vi "SMR_LabVIEW_V6.vi"() -> ()   [LabVIEW 2025]
uses:
  <vilib>/DAQmx/read.llb/DAQmx Read (Analog 1D DBL NChan 1Samp).vi
  <vilib>/DAQmx/create/channels.llb/DAQmx Create Channel (AI-Temperature-Thermocouple).vi
  <vilib>/DAQmx/create/channels.llb/DAQmx Create Channel (AI-Voltage-Basic).vi
  <vilib>/DAQmx/miscellaneous.llb/DAQmx Fill In Error Info.vi
panel:
  in  "Flow CSV Path":path
  in  "Pressure CSV Path":path
  in  "Temeprature CSV Path":path
  out "Heat Exchanger Pressure History":dbl(graph)
  out "Main Loop Pressure History":T1(graph)
  out "Heat Exchanger Temperature History":cluster{"Waveform":dbl, "Waveform":dbl}(graph)
  out "Main Loop Temeperature History":T2(graph)
  out "Overall Avg Pressure (psi)":dbl
  out "Heat Exchanger Pressure P6 (psi)":dbl
  out "Main Loop Avg Pressure (psi)":dbl
  out "Heat Exchanger Avg Temp (deg C)":dbl
  out "Main Loop Avg Temp (deg C)":dbl
  out "Raw NI9201 \nVoltage Display":T3
  out "Temperature Display":T4
  out "Pressure Display":T5
  in  "Flow Offset Correction (GPM)":dbl=-0.3
  out "Flow History":dbl(graph)
  out "Overall Pressure History":T6(graph)
  out "Overall Temperature History":T7(graph)
  out "Max Loop Pressure (psi)":dbl
  out "Overall Avg Temp (deg C)":dbl
  out "Max Loop Temp (deg C)":dbl
  out "Heat Exchanger Flow (GPM)":dbl
  in  "Loop Period (ms)":dbl=1000.0
  in  "Stop":bool
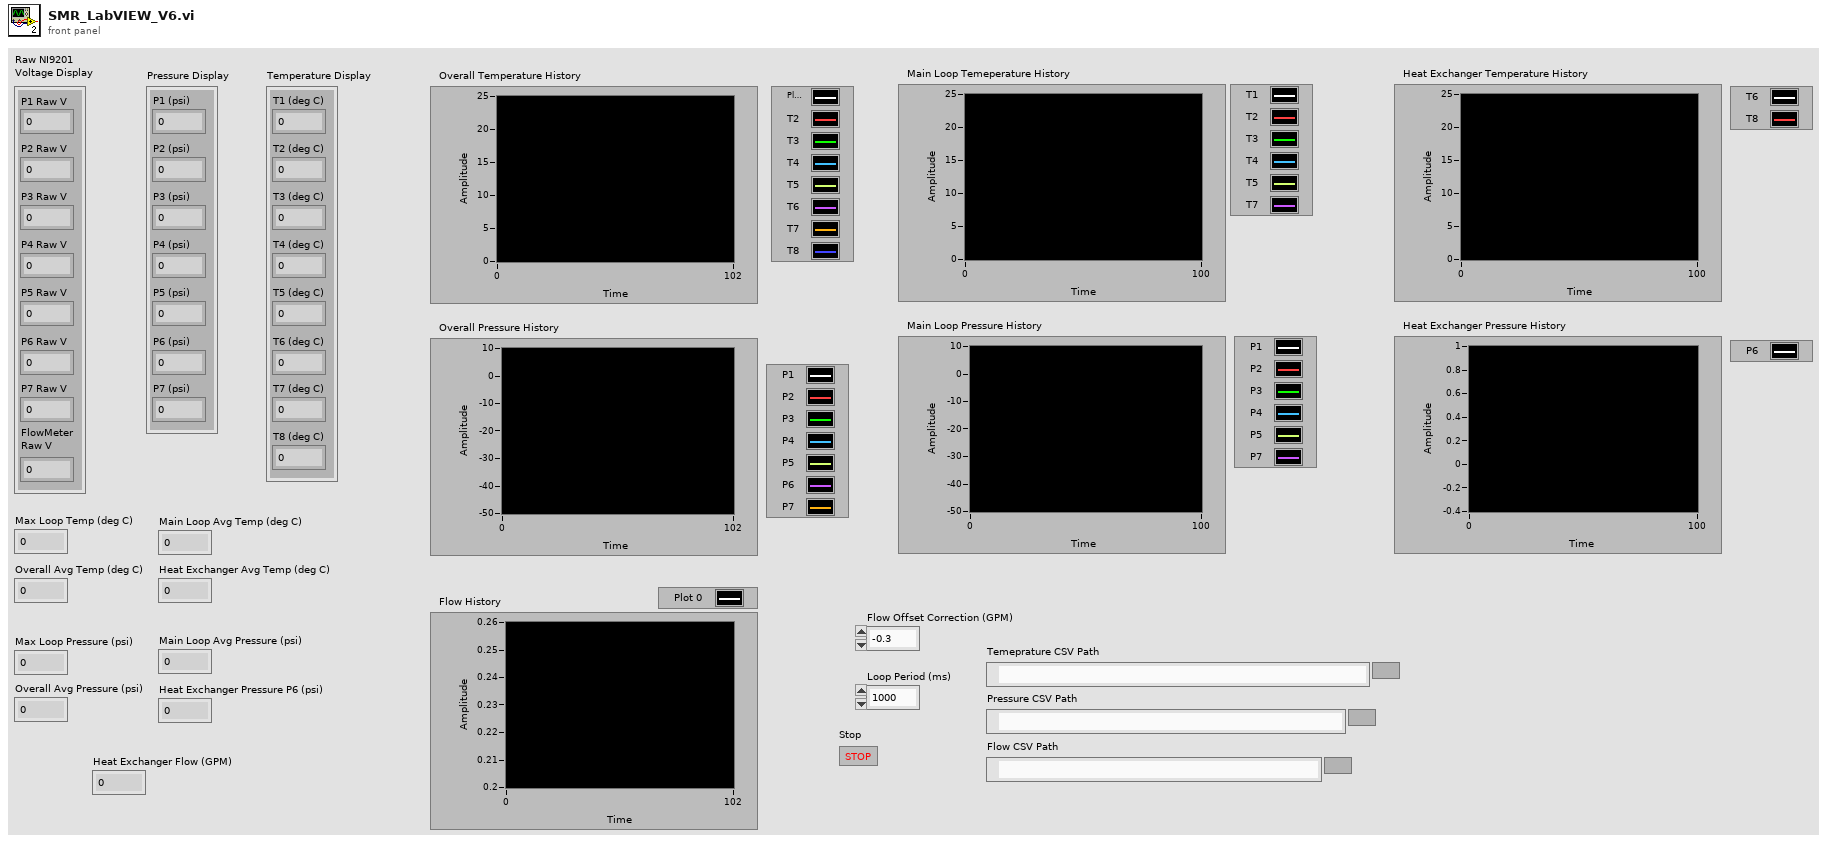
[diagram p1: front panel]
types:
  T1 = cluster{"P1":dbl, "P2":dbl, "P3":dbl, "P4":dbl, "P5":dbl, "P7":dbl}
  T2 = cluster{"Waveform":dbl, "Waveform":dbl, "Waveform":dbl, "Waveform":dbl, "Waveform":dbl, "Waveform":dbl}
  T3 = cluster{"P1 Raw V":dbl, "P2 Raw V":dbl, "P3 Raw V":dbl, "P4 Raw V":dbl, "P5 Raw V":dbl, "P6 Raw V":dbl, "P7 Raw V":dbl, "FlowMeter\nRaw V":dbl}
  T4 = cluster{"T1 (deg C)":dbl, "T2 (deg C)":dbl, "T3 (deg C)":dbl, "T4 (deg C)":dbl, "T5 (deg C)":dbl, "T6 (deg C)":dbl, "T7 (deg C)":dbl, "T8 (deg C)":dbl}
  T5 = cluster{"P1 (psi)":dbl, "P2 (psi)":dbl, "P3 (psi)":dbl, "P4 (psi)":dbl, "P5 (psi)":dbl, "P6 (psi)":dbl, "P7 (psi)":dbl}
  T6 = cluster{"P1":dbl, "P2":dbl, "P3":dbl, "P4":dbl, "P5":dbl, "P6":dbl, "P7":dbl}
  T7 = cluster{"Waveform":dbl, "Waveform":dbl, "Waveform":dbl, "Waveform":dbl, "Waveform":dbl, "Waveform":dbl, "Waveform":dbl, "Waveform":dbl}
  T8 = enum16{"open", "replace", "create", "open or create", "replace or create", "replace or create with confirmation"}
  T9 = cluster{"P1":dbl, "P2":dbl, "P3":dbl, "P4":dbl, "P5":dbl, "P6":dbl, "P7":dbl, "Flow":dbl}
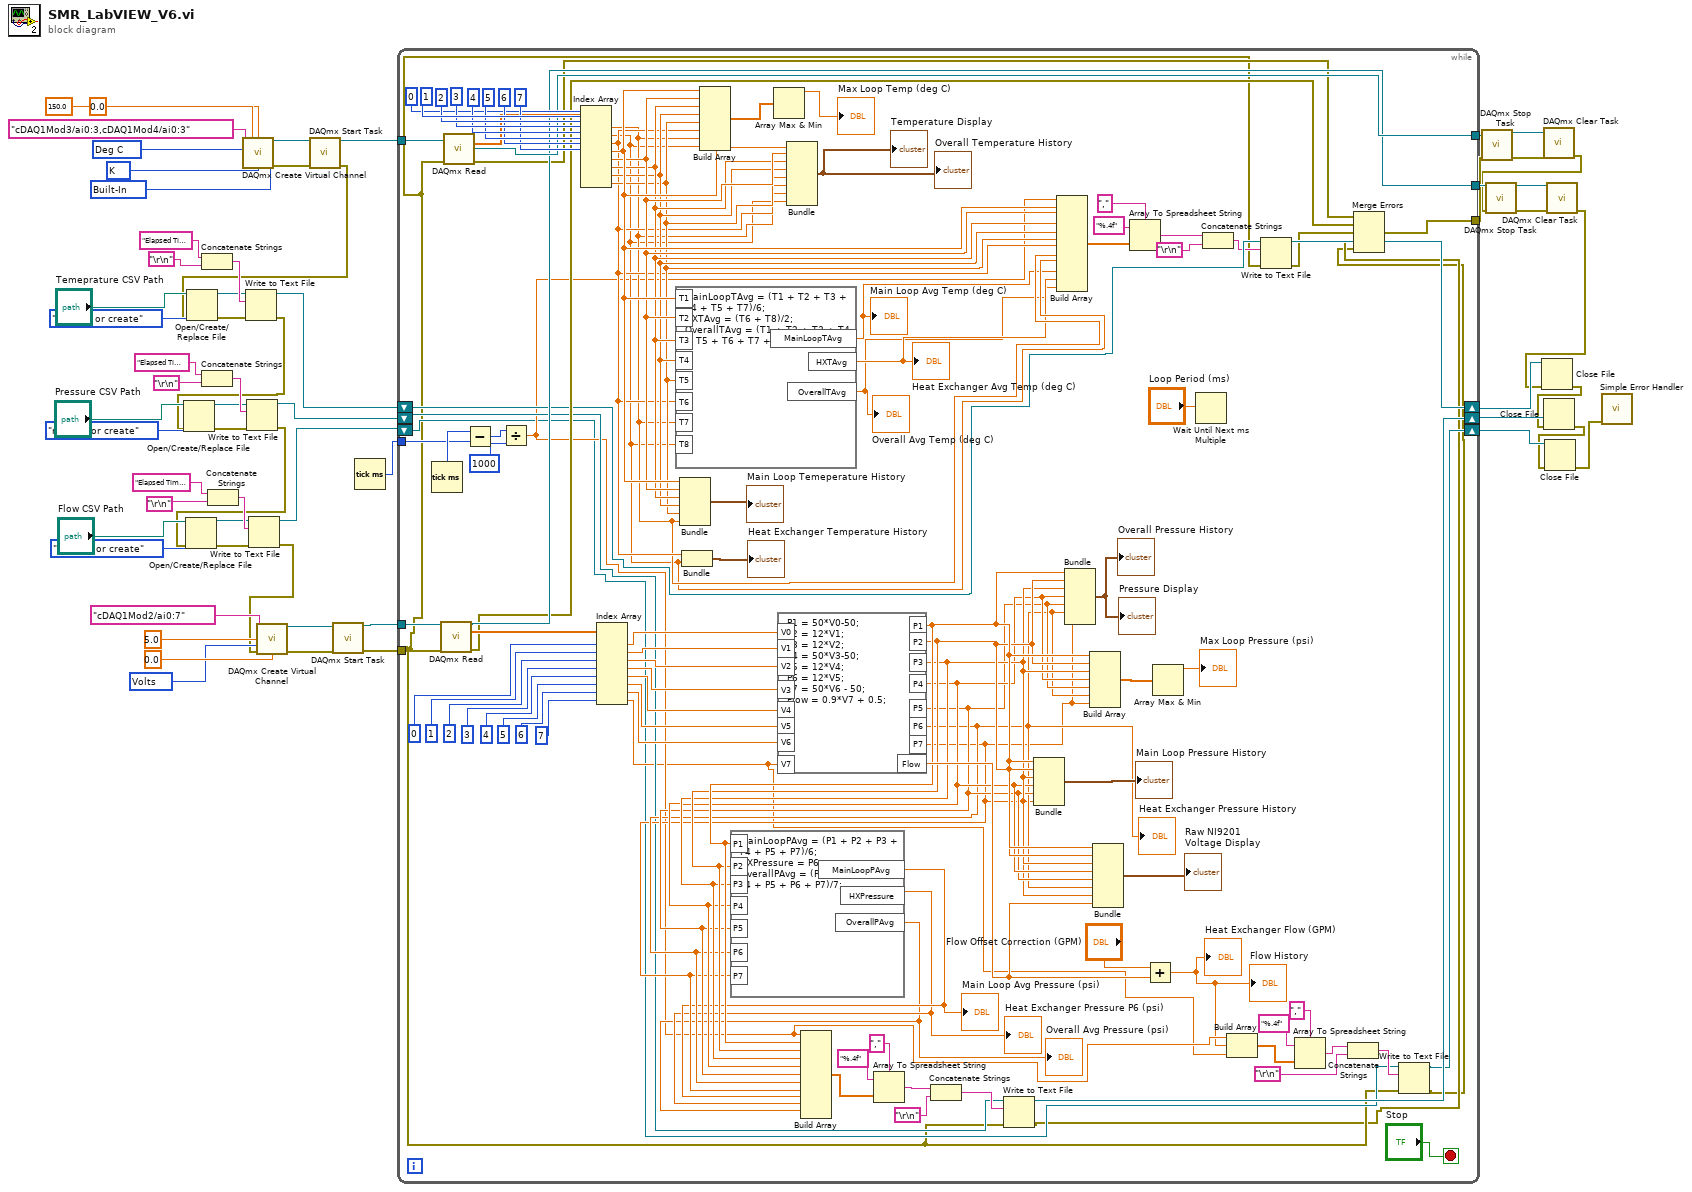
[diagram p0: block diagram]
diagram:
  w49 = 10200 items=["Built-In"=10200, "Constant Value"=10116, "Channel"=10113] ("cjc source")
  w50 = 10073 items=["J"=10072, "K"=10073, "N"=10077, "R"=10082, "S"=10085, "T"=10086, "B"=10047, "E"=10055] ("thermocouple type")
  w51 = 10143 items=["Deg C"=10143, "Deg F"=10144, "Kelvins"=10325, "Deg R"=10145, "From Custom Scale"=10065] ("units")
  w58 = 10348 items=["Volts"=10348, "From Custom Scale"=10065] ("units")
  n1 = Concatenate Strings("Elapsed Time (s),T1 (deg C),T2 (deg C),T3 (deg C),T4 (deg C),T5 (deg C),T6 (deg C),T7 (deg C),T8 (deg C),Main Loop Avg Temp (deg C),HX Avg Temp (deg C),Overall Avg Temp (deg C)", "\r\n") -> (w28:string)
  n2 = Concatenate Strings("Elapsed Time (s),P1 (psi),P2 (psi),P3 (psi),P4 (psi),P5 (psi),P6 (psi),P7 (psi),Main Loop Avg Pressure (psi),HX Pressure (psi),Overall Avg Pressure (psi)", "\r\n") -> (w26:string)
  n3 = Concatenate Strings("Elapsed Time (s),Heat Exchanger Flow (GPM),Flow Raw Voltage (V)", "\r\n") -> (w22:string)
  n4 = call-poly <vilib>:"DAQmx Create Virtual Channel.vi"("maximum value"=150.0, "minimum value"=0.0, "physical channels"=tag "cDAQ1Mod3/ai0:3,cDAQ1Mod4/ai0:3", "cjc source"=w49, "units"=w51, "thermocouple type"=w50) -> ("task out"=w48:refnum<k21>, "error out"=w47:errorcluster)  [unwired: 8 in]
  n5 = call <vilib>:"DAQmx Start Task.vi"("task/channels in"=w48, "error in"=w47) -> ("task out"=w46:refnum<k21>, "error out"=w11:errorcluster)  [unwired: 12 in]
  n6 = Open/Create/Replace File(file path (use dialog)="Temeprature CSV Path", error in=w11, operation (0:open)=T8."replace or create") -> (refnum out=w27:refnum<file>, error out=w10:errorcluster)  [unwired: 3 in, 1 out]
  n7 = Write to Text File(file (use dialog)=w27, text=w28, error in=w10) -> (refnum out=w18:refnum<file>, error out=w9:errorcluster)  [unwired: 1 in, 1 out]
  n8 = Open/Create/Replace File(file path (use dialog)="Pressure CSV Path", error in=w9, operation (0:open)=T8."replace or create") -> (refnum out=w25:refnum<file>, error out=w8:errorcluster)  [unwired: 3 in, 1 out]
  n9 = Write to Text File(file (use dialog)=w25, text=w26, error in=w8) -> (refnum out=w17:refnum<file>, error out=w7:errorcluster)  [unwired: 1 in, 1 out]
  n10 = Open/Create/Replace File(file path (use dialog)="Flow CSV Path", error in=w7, operation (0:open)=T8."replace or create") -> (refnum out=w21:refnum<file>, error out=w6:errorcluster)  [unwired: 3 in, 1 out]
  n11 = Write to Text File(file (use dialog)=w21, text=w22, error in=w6) -> (refnum out=w16:refnum<file>, error out=w5:errorcluster)  [unwired: 1 in, 1 out]
  n12 = call-poly <vilib>:"DAQmx Create Virtual Channel.vi"("maximum value"=5.0, "minimum value"=0.0, "physical channels"=tag "cDAQ1Mod2/ai0:7", "units"=w58, "error in"=w5) -> ("task out"=w57:refnum<k21>, "error out"=w56:errorcluster)  [unwired: 9 in]
  n13 = call <vilib>:"DAQmx Start Task.vi"("task/channels in"=w57, "error in"=w56) -> ("task out"=w55:refnum<k21>, "error out"=w44:errorcluster)  [unwired: 12 in]
  n14 = Tick Count (ms)() -> (millisecond timer value=w15:u32)
  n15 = while {
    tunnel: w55 -> [w159]
    tunnel: w46 -> [w132]
    tunnel: [w122] -> w45
    tunnel: w44 -> [w65]
    tunnel: [w121] -> w43
    tunnel: [w118] -> w42
    shift-right: [w96] -> w14
    shift-left: w18 -> [w97]
    shift-right: [w77] -> w13
    shift-left: w17 -> [w78]
    shift-right: [w66] -> w12
    shift-left: w16 -> [w67]
    tunnel: w15 -> [w116]
    stop <- "Stop" stop-if-true
    n16 = Tick Count (ms)() -> (millisecond timer value=w117:u32)
    n17 = call-poly <vilib>:"DAQmx Read.vi"("task/channels in"=w159, "error in"=w65) -> ("task out"=w121:refnum<k21>, "data"=w150:dbl[], "error out"=w119:errorcluster)  [unwired: 11 in]
    n18 = call-poly <vilib>:"DAQmx Read.vi"("task/channels in"=w132, "error in"=w65) -> ("task out"=w122:refnum<k21>, "data"=w123:dbl[], "error out"=w120:errorcluster)  [unwired: 11 in]
    n19 = Subtract(x=w117, y=w116) -> (x-y=w115:u32)
    n20 = Divide(x=w115, y=u32 1000) -> (x/y=w76:dbl)
    n21 = Index Array(array=w123, index #1=0 ("index"), index #2=1 ("index"), index #3=2 ("index"), index #4=3 ("index"), index #5=4 ("index"), index #6=5 ("index"), index #7=6 ("index"), index #8=7 ("index")) -> (element #1=w107:dbl, element #2=w106:dbl, element #3=w108:dbl, element #4=w113:dbl, element #5=w112:dbl, element #6=w111:dbl, element #7=w110:dbl, element #8=w109:dbl)
    n22 = Index Array(array=w150, index #1=0 ("index"), index #2=1 ("index"), index #3=2 ("index"), index #4=3 ("index"), index #5=4 ("index"), index #6=5 ("index"), index #7=6 ("index"), index #8=7 ("index")) -> (element #1=w149:dbl, element #2=w148:dbl, element #3=w147:dbl, element #4=w146:dbl, element #5=w145:dbl, element #6=w144:dbl, element #7=w143:dbl, element #8=w74:dbl)
    n23 = formula code="MainLoopTAvg = (T1 + T2 + T3 + T4 + T5 + T7)/6;\nHXTAvg = (T6 + T8)/2;\nOverallTAvg = (T1 + T2 + T3 + T4 + T5 + T6 + T7 + T8)/8;"("T1"=w113, "T2"=w112, "T3"=w111, "T4"=w110, "T5"=w109, "T6"=w108, "T7"=w107, "T8"=w106) -> ("MainLoopTAvg"=w105:dbl, "HXTAvg"=w104:dbl, "OverallTAvg"=w103:dbl)
    "Overall Avg Temp (deg C)" <- w103
    "Main Loop Avg Temp (deg C)" <- w105
    "Heat Exchanger Avg Temp (deg C)" <- w104
    n24 = Bundle("Waveform"=w113, "Waveform"=w112, "Waveform"=w111, "Waveform"=w110, "Waveform"=w109, "Waveform"=w107) -> (→"Main Loop Temeperature History":T2)  [unwired: 1 in]
    n25 = Bundle("Waveform"=w108, "Waveform"=w106) -> (→"Heat Exchanger Temperature History":cluster{"Waveform":dbl, "Waveform":dbl})  [unwired: 1 in]
    n26 = Build Array(w113, w112, w111, w110, w109, w108, w107, w106) -> (w160:dbl[])
    n27 = Array Max & Min(array=w160) -> (max value=→"Max Loop Temp (deg C)":dbl)  [unwired: 3 out]
    n28 = formula code="P1 = 50*V0-50;\nP2 = 12*V1;\nP3 = 12*V2;\nP4 = 50*V3-50;\nP5 = 12*V4;\nP6 = 12*V5; \nP7 = 50*V6 - 50;\nFlow = 0.9*V7 + 0.5;"("V0"=w149, "V1"=w148, "V2"=w147, "V3"=w146, "V4"=w145, "V5"=w144, "V6"=w143, "V7"=w74) -> ("P1"=w95:dbl, "P2"=w94:dbl, "P3"=w93:dbl, "P4"=w92:dbl, "P5"=w91:dbl, "P6"=w90:dbl, "P7"=w89:dbl, "Flow"=w137:dbl)
    "Heat Exchanger Pressure History" <- w90
    n29 = formula code="MainLoopPAvg = (P1 + P2 + P3 + P4 + P5 + P7)/6;\nHXPressure = P6;\nOverallPAvg = (P1 + P2 + P3 + P4 + P5 + P6 + P7)/7;"("P1"=w95, "P2"=w94, "P3"=w93, "P4"=w92, "P5"=w91, "P6"=w90, "P7"=w89) -> ("MainLoopPAvg"=w88:dbl, "HXPressure"=w87:dbl, "OverallPAvg"=w86:dbl)
    "Overall Avg Pressure (psi)" <- w86
    "Heat Exchanger Pressure P6 (psi)" <- w87
    "Main Loop Avg Pressure (psi)" <- w88
    n30 = Bundle("Waveform"=w113, "Waveform"=w112, "Waveform"=w111, "Waveform"=w110, "Waveform"=w109, "Waveform"=w108, "Waveform"=w107, "Waveform"=w106) -> (→"Overall Temperature History" →"Temperature Display":T7)  [unwired: 1 in]
    n31 = Build Array(w76, w95, w94, w93, w92, w91, w90, w89, w88, w87, w86) -> (w85:dbl[])
    n32 = Array To Spreadsheet String(delimiter (Tab)=",", array=w85, 3:"%.4f" ("format string")) -> (spreadsheet string=w81:string)
    n33 = Concatenate Strings(w81, "\r\n") -> (w79:string)
    n34 = Write to Text File(file (use dialog)=w78, text=w79, error in=w65) -> (refnum out=w77:refnum<file>, error out=w63:errorcluster)  [unwired: 1 in, 1 out]
    n35 = Bundle("P1"=w95, "P2"=w94, "P3"=w93, "P4"=w92, "P5"=w91, "P7"=w89) -> (→"Main Loop Pressure History":T1)  [unwired: 1 in]
    n36 = Build Array(w76, w113, w112, w111, w110, w109, w108, w107, w106, w105, w104, w103) -> (w102:dbl[])
    n37 = Bundle("P1"=w95, "P2"=w94, "P3"=w93, "P4"=w92, "P5"=w91, "P6"=w90, "P7"=w89) -> (→"Overall Pressure History" →"Pressure Display":T6)  [unwired: 1 in]
    n38 = Build Array(w95, w94, w93, w92, w91, w90, w89) -> (w140:dbl[])
    n39 = Bundle("P1"=w95, "P2"=w94, "P3"=w93, "P4"=w92, "P5"=w91, "P6"=w90, "P7"=w89, "Flow"=w137) -> (→"Raw NI9201 \nVoltage Display":T9)  [unwired: 1 in]
    n40 = Array To Spreadsheet String(delimiter (Tab)=",", array=w102, 3:"%.4f" ("format string")) -> (spreadsheet string=w99:string)
    n41 = Add(x="Flow Offset Correction (GPM)", y=w137) -> (x+y=w75:dbl)
    "Heat Exchanger Flow (GPM)" <- w75
    "Flow History" <- w75
    n42 = Array Max & Min(array=w140) -> (max value=→"Max Loop Pressure (psi)":dbl)  [unwired: 3 out]
    n43 = Wait Until Next ms Multiple(millisecond multiple="Loop Period (ms)") -> ()  [unwired: 1 out]
    n44 = Concatenate Strings(w99, "\r\n") -> (w82:string)
    n45 = Build Array(w76, w75, w74) -> (w73:dbl[])
    n46 = Write to Text File(file (use dialog)=w97, text=w82, error in=w65) -> (refnum out=w96:refnum<file>, error out=w64:errorcluster)  [unwired: 1 in, 1 out]
    n47 = Array To Spreadsheet String(delimiter (Tab)=",", array=w73, 3:"%.4f" ("format string")) -> (spreadsheet string=w69:string)
    n48 = Concatenate Strings(w69, "\r\n") -> (w68:string)
    n49 = Write to Text File(file (use dialog)=w67, text=w68, error in=w65) -> (refnum out=w66:refnum<file>, error out=w62:errorcluster)  [unwired: 1 in, 1 out]
    n50 = Merge Errors(w120, w119, w64, w63, w62) -> (w118:errorcluster)
  }
  n51 = call <vilib>:"DAQmx Stop Task.vi"("task/channels in"=w45, "error in"=w42) -> ("task out"=w41:refnum<k21>, "error out"=w39:errorcluster)  [unwired: 12 in]
  n52 = call <vilib>:"DAQmx Clear Task.vi"("task in"=w41, "error in"=w39) -> ("error out"=w38:errorcluster)  [unwired: 13 in]
  n53 = call <vilib>:"DAQmx Stop Task.vi"("task/channels in"=w43, "error in"=w38) -> ("task out"=w40:refnum<k21>, "error out"=w37:errorcluster)  [unwired: 12 in]
  n54 = call <vilib>:"DAQmx Clear Task.vi"("task in"=w40, "error in"=w37) -> ("error out"=w4:errorcluster)  [unwired: 13 in]
  n55 = Close File(refnum=w14, error in=w4) -> (error out=w3:errorcluster)  [unwired: 1 out]
  n56 = Close File(refnum=w13, error in=w3) -> (error out=w2:errorcluster)  [unwired: 1 out]
  n57 = Close File(refnum=w12, error in=w2) -> (error out=w1:errorcluster)  [unwired: 1 out]
  n58 = call <vilib>:"Simple Error Handler.vi"("error in (no error)"=w1) -> ()  [unwired: 4 in, 5 out]
